vi "Simple_OK-Warning_Prompt-W.vi"(3 "error in":errorcluster, 4 "User Message In":string="Range values for base size in inches are : 0 to 16.00\nMinimum and maximum values in milimeters are: 0 to 400", 5 "Panel In":refnum<class "Panel.lvclass">) -> (0 "error out":errorcluster, 1 "OK Button":bool)   [LabVIEW 2023]
uses:
  <vilib>/MGI/Panel Manager/Panel/Panel/Panel.lvclass
  <userlib>/_OpenG.lib/appcontrol/appcontrol.llb/openg_application_control.lvlib
panel:
  in  "OK Button":bool
  out "User Message Out":string
  in  "Close Button":bool
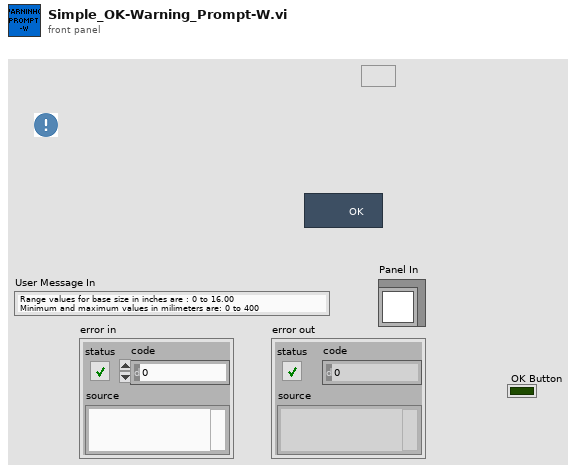
[diagram p1: front panel]
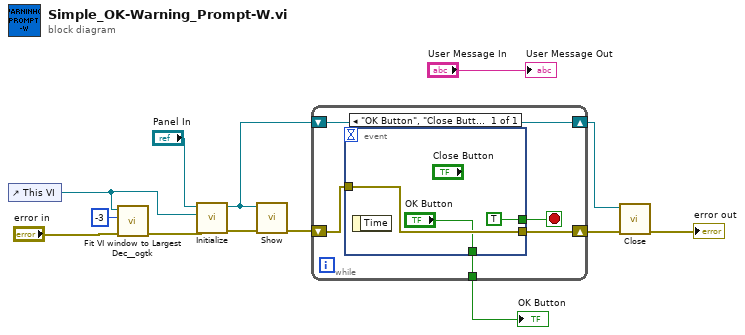
[diagram p0: block diagram]
diagram:
  n1 = control-ref of="This VI"() -> (w3:refnum<vi>)
  n2 = call <userlib>:"Fit VI window to Largest Dec__ogtk.vi"("error in (no error)"="error in", "border spacing (2 px)"=-3, "VI Ref (calling VI)"=w3) -> ("error out"=w9:errorcluster)  [unwired: 3 in, 1 out]
  n3 = call <vilib>:"Initialize.vi"("error in (no error)"=w9, "VI Refnum"=w3, "Panel In"="Panel In") -> ("error out"=w8:errorcluster, "Panel Out"=w4:refnum<class "Panel.lvclass">)  [unwired: 6 in, 1 out]
  n4 = call <vilib>:"Show.vi"("Error In"=w8, "Panel in"=w4) -> ("Error Out"=w5:errorcluster)  [unwired: 9 in]
  n5 = while {
    shift-right: [w16] -> w11
    shift-left: w5 -> [w17]
    shift-right: [w15] -> w6
    shift-left: w4 -> [w15]
    tunnel: [w14] -> w1
    stop <- w18 stop-if-true
    n6 = event shown="[0] \"OK Button\", \"Close Button\": Value Change" {
      selector: _ -> [_]
      dyn-events: _ -> [_]
      timeout: _ -> [_]
      tunnel: [TRUE] -> w18
      tunnel: w17 -> [w20]
      tunnel: [w20] -> w16
      tunnel: ["OK Button"] -> w14
      event "OK Button", "Close Button": Value Change {
        n7 = event-data() -> ()  [unwired: 1 in, 1 out]
      }
    }
  }
  "OK Button" <- w1
  n8 = call-dynamic "Close.vi"("Error In"=w11, "Panel In"=w6) -> ("Error Out"=→"error out":errorcluster)  [unwired: 9 in]
  "User Message Out" <- "User Message In"
